vi "HalfWavePlate.vi"(0 "VISA":T1={"Resource Name"="COM6", "Init VISA"=TRUE, "Close VISA"=TRUE, "VISA or TCP/IP"=FALSE, "IP Address/Hostname"="10.21.163.30"}, 1 "Degrees":dbl=500.0, 2 "Motor":dbl min=0.0 max=1.0 step=1.0) -> ()   [LabVIEW 2016]
uses:
  Misc/Intelligent Picomotor Driver/Example_LabVIEW 6.1_MCL Rev E.llb/VISA & TCPIP Control.ctl
panel:
  in  "Conversion factor\n(input #/degrees)":dbl=44.0
  # "Motor 0: Overall trap power\n\nMotor 1: Differential trap power"
  # "This value was measured\nfor motor 1 on 150219. It\nisn't exact."
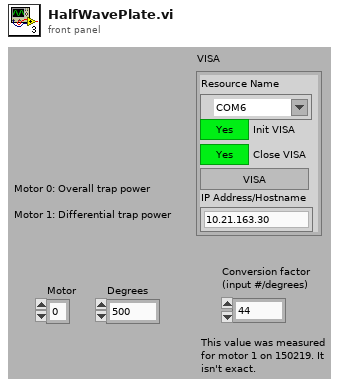
[diagram p1: front panel]
types:
  T1 = typedef "VISA & TCPIP Control.ctl" = cluster{"Resource Name":refnum<visa-resource-name>, "Init VISA":bool, "Close VISA":bool, "VISA or TCP/IP":bool, "IP Address/Hostname":string}
  T2 = typedef "Error.ctl" = errorcluster
  T3 = typedef "Pico Motor Status Byte.ctl" = cluster{"Moving":bool, "Check Sum Err":bool, "Motor On":bool, "Motor Selector":bool, "At Cmd Velocity":bool, "Velocity Mode":bool, "Position Profile Mode":bool, "Reserved":bool}
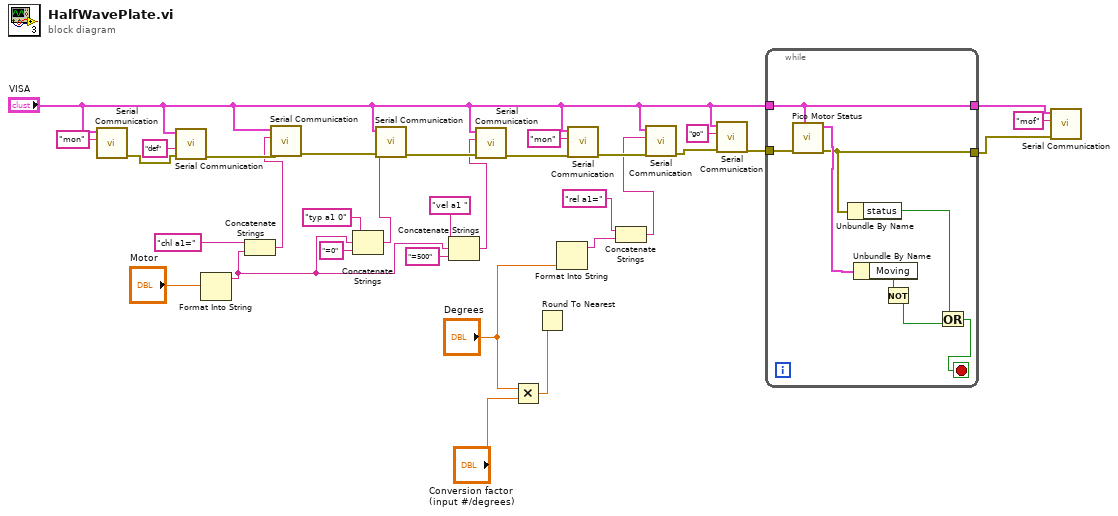
[diagram p0: block diagram]
diagram:
  n1 = call "Serial Communication.vi"("Write String"="mon", "VISA"="VISA") -> ("Error Out"=w28:T2)  [unwired: 8 in, 1 out]
  n2 = call "Serial Communication.vi"("Error In (no error)"=w28, "Write String"="def", "VISA"="VISA") -> ("Error Out"=w27:T2)  [unwired: 7 in, 1 out]
  n3 = Format Into String("Motor") -> (resulting string=w13:string)  [unwired: 3 in, 1 out]
  n4 = Concatenate Strings("chl a1=" ("Write String"), w13) -> (w20:string)
  n5 = call "Serial Communication.vi"("Error In (no error)"=w27, "Write String"=w20, "VISA"="VISA") -> ("Error Out"=w26:T2)  [unwired: 7 in, 1 out]
  n6 = Concatenate Strings("typ a1 0" ("Write String"), w13, "=0" ("string")) -> (w15:string)
  n7 = call "Serial Communication.vi"("Error In (no error)"=w26, "Write String"=w15, "VISA"="VISA") -> ("Error Out"=w25:T2)  [unwired: 7 in, 1 out]
  n8 = Concatenate Strings("vel a1 " ("Write String"), w13, "=500" ("string")) -> (w12:string)
  n9 = call "Serial Communication.vi"("Error In (no error)"=w25, "Write String"=w12, "VISA"="VISA") -> ("Error Out"=w24:T2)  [unwired: 7 in, 1 out]
  n10 = Multiply(x="Degrees", y="Conversion factor\n(input #/degrees)") -> (x*y=w2:dbl)
  n11 = Round To Nearest(number=w2) -> ()  [unwired: 1 out]
  n12 = Format Into String("Degrees") -> (resulting string=w10:string)  [unwired: 3 in, 1 out]
  n13 = call "Serial Communication.vi"("Error In (no error)"=w24, "Write String"="mon", "VISA"="VISA") -> ("Error Out"=w23:T2)  [unwired: 7 in, 1 out]
  n14 = Concatenate Strings("rel a1=" ("Write String"), w10) -> (w9:string)
  n15 = call "Serial Communication.vi"("Error In (no error)"=w23, "Write String"=w9, "VISA"="VISA") -> ("Error Out"=w22:T2)  [unwired: 7 in, 1 out]
  n16 = call "Serial Communication.vi"("Error In (no error)"=w22, "Write String"="go", "VISA"="VISA") -> ("Error Out"=w8:T2)  [unwired: 7 in, 1 out]
  n17 = while {
    tunnel: w8 -> [w40]
    tunnel: "VISA" -> [w34]
    tunnel: [w34] -> w5
    tunnel: [w33] -> w6
    stop <- w35 stop-if-true
    n18 = call "Pico Motor Status.vi"("VISA"=w34, "error in"=w40) -> ("error out"=w33:T2, "Pico Status Byte"=w37:T3)  [unwired: 8 in]
    n19 = Unbundle By Name(w33) -> ("status"=w39:bool)
    n20 = Unbundle By Name(w37) -> ("Moving"=w36:bool)
    n21 = Not(x=w36) -> (.not. x?=w38:bool)
    n22 = Or(x=w39, y=w38) -> (x .or. y?=w35:bool)
  }
  n23 = call "Serial Communication.vi"("Error In (no error)"=w6, "Write String"="mof", "VISA"=w5) -> ()  [unwired: 7 in, 2 out]
